vi "Store Configuration Parameters.vi"(8 "error in (no error)":errorcluster, 10 "refnum":T1, 11 "Example Configuration Dialog in":refnum<class "GaugeController Configuration.lvclass">) -> (0 "error out":errorcluster, 2 "refnum out":T1, 3 "Example Configuration Dialog out":refnum<class "GaugeController Configuration.lvclass">)   [LabVIEW 2016, in "Hardware.lvlib" / "GaugeController.lvlib" / "GaugeController Configuration.lvclass"]
uses:
  <userlib>/Common Components/Hardware/GaugeController/GaugeController Config/GaugeController Configuration.lvclass
  <vilib>/Utility/config.llb/Config Data RefNum.ctl
  <userlib>/Common Components/Hardware/GaugeController/GaugeController Config/GaugeController Configuration.lvclass/GaugeController Configuration.ctl
  <userlib>/Common Components/Hardware/Abstract Hardware/Hardware.lvclass/Hardware.ctl
  <userlib>/Common Components/Hardware/DevInfo/DevInfo.lvclass/DevInfo.ctl
  <userlib>/Common Components/Hardware/GaugeController/GaugeController Config/Accessors/Read GaugeController Obj.vi
  <userlib>/Common Components/Hardware/Abstract Hardware/Read Label.vi
  <userlib>/Common Components/Hardware/Abstract Hardware/Read DevInfo.vi
  <userlib>/Common Components/Hardware/DevInfo/Read HW Type.vi
  <userlib>/Common Components/Hardware/DevInfo/Read Device Name.vi
  <userlib>/Common Components/Hardware/DevInfo/Read COMM Address.vi
  <userlib>/Common Components/Hardware/DevInfo/Read Sub-COMM Address.vi
  <userlib>/Common Components/Hardware/GaugeController/GaugeController/GaugeController.lvclass
  C:/Program Files (x86)/National Instruments/LabVIEW 2016/user.lib/Common Components/Hardware/Abstract Hardware/Hardware.lvclass
  <userlib>/Configuration Dialog Actor/Configuration.lvclass
  <userlib>/Common Components/Hardware/DevInfo/DevInfo.lvclass
  <vilib>/Utility/config.llb/NI_LVConfig.lvlib
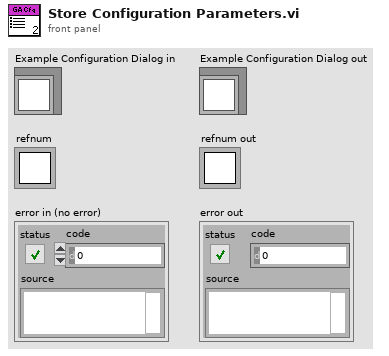
[diagram p1: front panel]
types:
  T1 = typedef "NI_LVConfig.lvlib/Config Data RefNum.ctl" = refnum<k1>
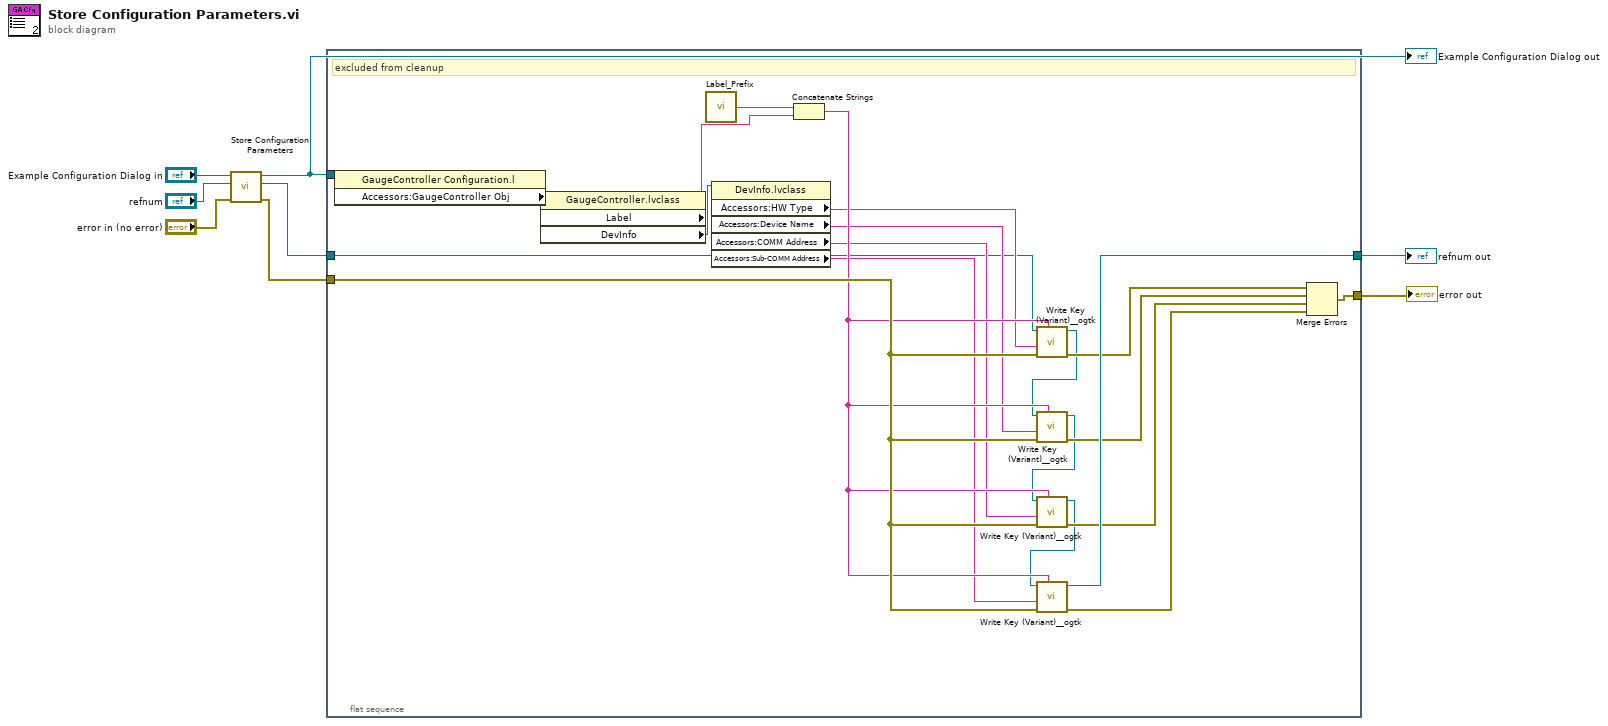
[diagram p0: block diagram]
diagram:
  n1 = call-parent "Store Configuration Parameters.vi"("error in (no error)"="error in (no error)", "refnum"="refnum", "Configuration in"="Example Configuration Dialog in") -> ("error out"=w4:errorcluster, "refnum out"=w5:T1, "Configuration out"=w3:refnum<class "GaugeController Configuration.lvclass">)  [unwired: 6 in]
  "Example Configuration Dialog out" <- w3
  n2 = flat-sequence {
    tunnel: w5 -> [w9]
    tunnel: w4 -> [w29]
    tunnel: w3 -> [w28]
    tunnel: [w27] -> w2
    tunnel: [w26] -> w1
    frame #0 {
      # "excluded from cleanup"
      n3 = property class="GaugeController Configuration.l"(reference=w28) -> ("Accessors:GaugeController Obj"=w14:refnum<class "GaugeController.lvclass">)  [unwired: 1 in, 2 out]
      n4 = property class="GaugeController.lvclass"(reference=w14) -> ("Label"=w16:string, "DevInfo"=w15:refnum<class "DevInfo.lvclass">)  [unwired: 1 in, 2 out]
      n5 = call <userlib>:"Label_Prefix.vi"() -> ("Label Prefix String"=w25:string)
      n6 = property class="DevInfo.lvclass"(reference=w15) -> ("Accessors:HW Type"=w13:string, "Accessors:Device Name"=w12:string, "Accessors:COMM Address"=w11:string, "Accessors:Sub-COMM Address"=w10:string)  [unwired: 1 in, 2 out]
      n7 = Concatenate Strings(w25, w16) -> (w24:string)
      n8 = call <userlib>:"Write Key (Variant)__ogtk.vi"("section"=w24, "error in (no error)"=w29, "key-value"=w13, "refnum"=w9) -> ("error out"=w23:errorcluster, "refnum out"=w19:T1)  [unwired: 6 in]
      n9 = call <userlib>:"Write Key (Variant)__ogtk.vi"("section"=w24, "error in (no error)"=w29, "key-value"=w12, "refnum"=w19) -> ("error out"=w22:errorcluster, "refnum out"=w18:T1)  [unwired: 6 in]
      n10 = call <userlib>:"Write Key (Variant)__ogtk.vi"("section"=w24, "error in (no error)"=w29, "key-value"=w11, "refnum"=w18) -> ("error out"=w21:errorcluster, "refnum out"=w17:T1)  [unwired: 6 in]
      n11 = call <userlib>:"Write Key (Variant)__ogtk.vi"("section"=w24, "error in (no error)"=w29, "key-value"=w10, "refnum"=w17) -> ("error out"=w20:errorcluster, "refnum out"=w27:T1)  [unwired: 6 in]
      n12 = Merge Errors(w23, w22, w21, w20) -> (w26:errorcluster)
    }
  }
  "error out" <- w1
  "refnum out" <- w2
